vi "Wait on Listener.vi"(8 "error in":errorcluster, 10 "timeout ms (wait forever: -1)":i32, 11 "TCP slave in":refnum<class "TCP Slave.lvclass">) -> (0 "error out":errorcluster, 1 "Timed Out":bool, 2 "connection reference":refnum<data-value>, 3 "TCP slave out":refnum<class "TCP Slave.lvclass">)   [LabVIEW 2013, in "Modbus Library - Advance.lvlib" / "TCP Slave.lvclass"]
doc: "Wrapper for the wait on listener VI, using the listener stored in the slave and an infinite timeout. When a connection is established, the output class will contain the new connection."
uses:
  TCP Slave.lvclass
  Connection.ctl
  TCP Slave.lvclass/TCP Slave.ctl
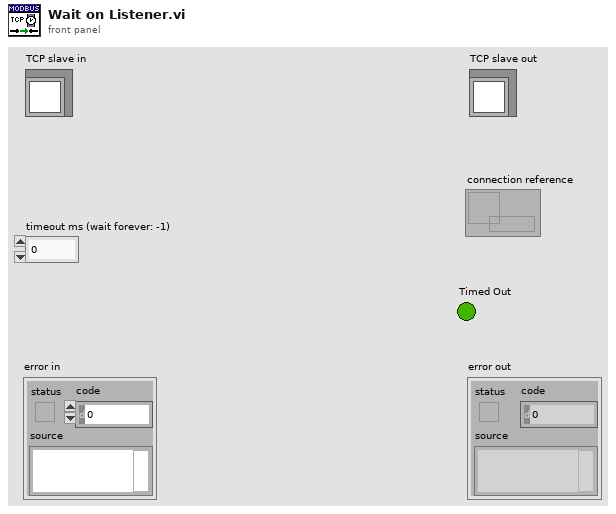
[diagram p1: front panel]
types:
  T1 = typedef "Modbus Library - Advance.lvlib/TCP Slave.lvclass/Connection.ctl" = cluster{"Connected?":bool, "IP address":string, "Port":u16, "connection error":errorcluster}
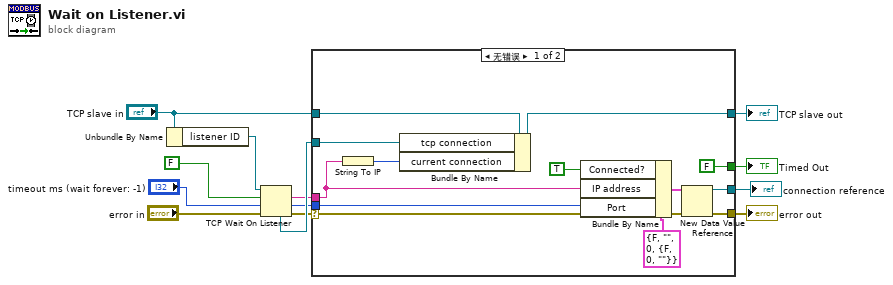
[diagram p0: block diagram]
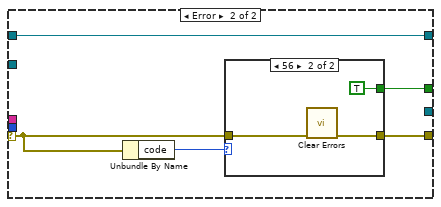
[diagram p2: hidden frame]
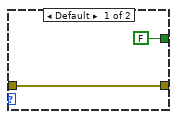
[diagram p3: hidden frame]
diagram:
  n1 = Unbundle By Name("TCP slave in") -> ("listener ID"=w11:refnum<k5>)
  n2 = TCP Wait On Listener(8:"error in", 9:"timeout ms (wait forever: -1)", 10:FALSE ("resolve remote address (T)"), 11:w11) -> (0:w6:errorcluster, 1:w1:u16, 2:w2:string, 4:w10:refnum<k5>)  [unwired: 1 out]
  n3 = case shown="无错误" w6 {
    selector: w6 -> [w22 w30]
    tunnel: "TCP slave in" -> [w26 w27]
    tunnel: w10 -> [w25 _]
    tunnel: [w23 w27] -> w7
    tunnel: [w17 w29] -> w5
    tunnel: [FALSE w28] -> w4
    tunnel: [w21 _] -> w3
    tunnel: w2 -> [w16 _]
    tunnel: w1 -> [w14 _]
    frame No Error {
      n4 = String To IP(1:w16) -> (0:w15:u32)
      n5 = Bundle By Name(cluster=w26, "tcp connection"=w25, "current connection"=w15) -> (w23:refnum<class "TCP Slave.lvclass">)
      n6 = Bundle By Name(cluster=T1 {"Connected?"=FALSE, "IP address"="", "Port"=0, "connection error"={"status"=FALSE, "code"=0, "source"=""}} ("Connection"), "Connected?"=TRUE, "IP address"=w16, "Port"=w14) -> (w19:T1)
      n7 = New Data Value Reference(data value=w19, error in=w22) -> (data value reference=w21:refnum<data-value>, error out=w17:errorcluster)
    }
    frame Error {
      n8 = Unbundle By Name(w30) -> ("code"=w31:i32)
      n9 = case shown="56" w31 {
        tunnel: w30 -> [w33 w36]
        tunnel: [w33 w35] -> w29
        tunnel: [FALSE TRUE] -> w28
        frame Default {
        }
        frame 56 {
          n10 = call <vilib>:"Clear Errors.vi"("error in (no error)"=w36) -> ("error out"=w35:errorcluster)  [unwired: 6 in]
        }
      }
    }
  }
  "error out" <- w5
  "Timed Out" <- w4
  "connection reference" <- w3
  "TCP slave out" <- w7
